vi "1553B_Mode.vi"(10 "模式命令":u16=17 format="%.0b", 11 "RT地址":u16) -> (3 "1553B指令":string)   [LabVIEW 2012]
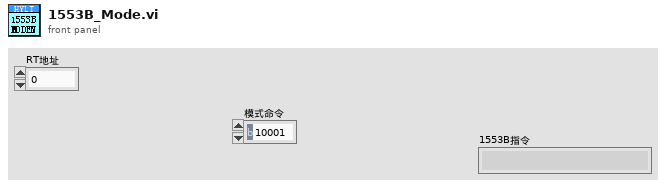
[diagram p1: front panel]
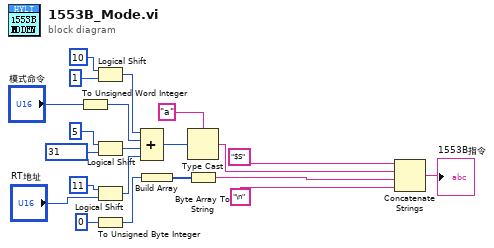
[diagram p0: block diagram]
diagram:
  n1 = To Unsigned Word Integer(number="模式命令") -> (unsigned 16bit integer=w2:u16)
  n2 = Logical Shift(y=u16 10, x=u16 1) -> (x << y=w3:u16)
  n3 = Logical Shift(y=i16 5, x=u16 31 ("子地址(默认：11111)")) -> (x << y=w1:u16)
  n4 = Logical Shift(y=i16 11, x="RT地址") -> (x << y=w16:u16)
  n5 = To Unsigned Byte Integer(number=u8 0 ("数字")) -> (unsigned 8bit integer=w9:u8)
  n6 = Compound Arithmetic op=ADD(w3, w2, w1, w16) -> (w15:u16)
  n7 = Build Array(w9) -> (w10:u8[])
  n8 = Type Cast(type="a" ("类型"), x=w15) -> (*(type *) &x=w14:string)
  n9 = Byte Array To String(unsigned byte array=w10) -> (string=w8:string)
  n10 = Concatenate Strings("$S" ("字符串"), w14, w8, "\n" ("字符串")) -> (→"1553B指令":string)
